vi "GetDataQDCV965A.vi"(8 "error in (no error)":errorcluster, 9 "#samples":i32=18, 10 "handle in":i32, 11 "VME module Base Address":u32) -> (0 "error out":errorcluster, 1 "Time Elapsed":u16, 2 "handle out":i32, 3 "Data":u32[](array[numeric]))   [LabVIEW 2014]
uses:
  Program Files (x86)/CAEN/Comm/labview/CAENComm.lvlib
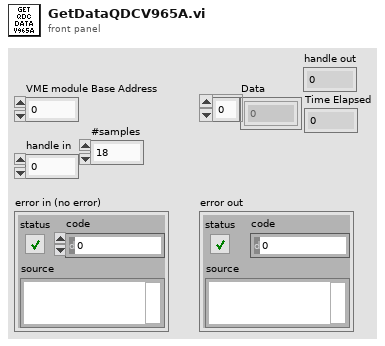
[diagram p1: front panel]
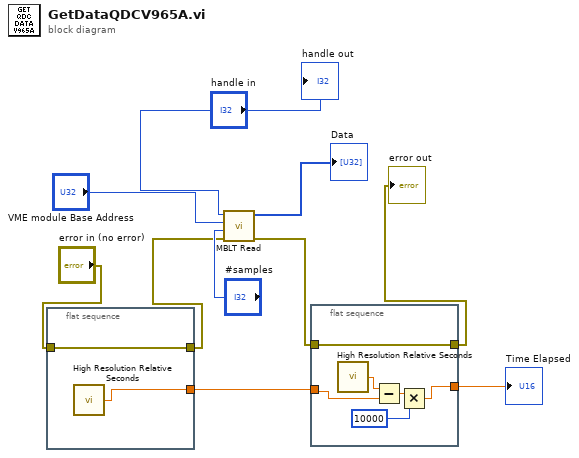
[diagram p0: block diagram]
diagram:
  n1 = flat-sequence {
    tunnel: "error in (no error)" -> [w12]
    tunnel: [w12] -> w3
    tunnel: [w11] -> w2
    frame #0 {
      n2 = call <vilib>:"High Resolution Relative Seconds.vi"() -> ("relative seconds"=w11:dbl)
    }
  }
  n3 = call "MBLT Read.vi"("error in (no error)"=w3, "BltSize"="#samples", "Address"="VME module Base Address", "handle"="handle in") -> ("error out"=w6:errorcluster, "Buff"=→"Data":u32[])  [unwired: 5 in, 1 out]
  n4 = flat-sequence {
    tunnel: w6 -> [w18]
    tunnel: [w18] -> w5
    tunnel: [w13] -> w1
    tunnel: w2 -> [w16]
    frame #0 {
      n5 = call <vilib>:"High Resolution Relative Seconds.vi"() -> ("relative seconds"=w17:dbl)
      n6 = Subtract(x=w17, y=w16) -> (x-y=w15:dbl)
      n7 = Multiply(x=w15, y=u16 10000) -> (x*y=w13:dbl)
    }
  }
  "error out" <- w5
  "handle out" <- "handle in"
  "Time Elapsed" <- w1
